vi "Segment File.vi"(8 "error in (no error)":errorcluster, 9 "current time in":timestamp, 10 "Current Bytes in":u64, 11 "Compiled.Settings":T1 {"Trigger Ref" format="%.0x"; "File Data"."Groups"."Channels"."Data Reference in" format="%.0x"}) -> (0 "error out":errorcluster, 1 "current time out":timestamp, 2 "Current Bytes out":u64, 3 "Boolean":bool)   [LabVIEW 2023, in "Embedded TDMS Logger Engine.lvlib"]
uses:
  Embedded TDMS Logger Engine.lvlib
  Shared/Compiled.Settings.ctl
  Shared/FileData.ctl
  Shared/GroupData.ctl
  Shared/Meta Data Item.ctl
  Shared/ChannelData.ctl
  <vilib>/NI VeriStand/Custom Device API/Data Reference.ctl
  Shared/SegmentOptions.ctl
  Shared/Embedded TDMS Logger Shared.lvlib
  <vilib>/NI VeriStand/Custom Device API/Custom Device API.lvlib
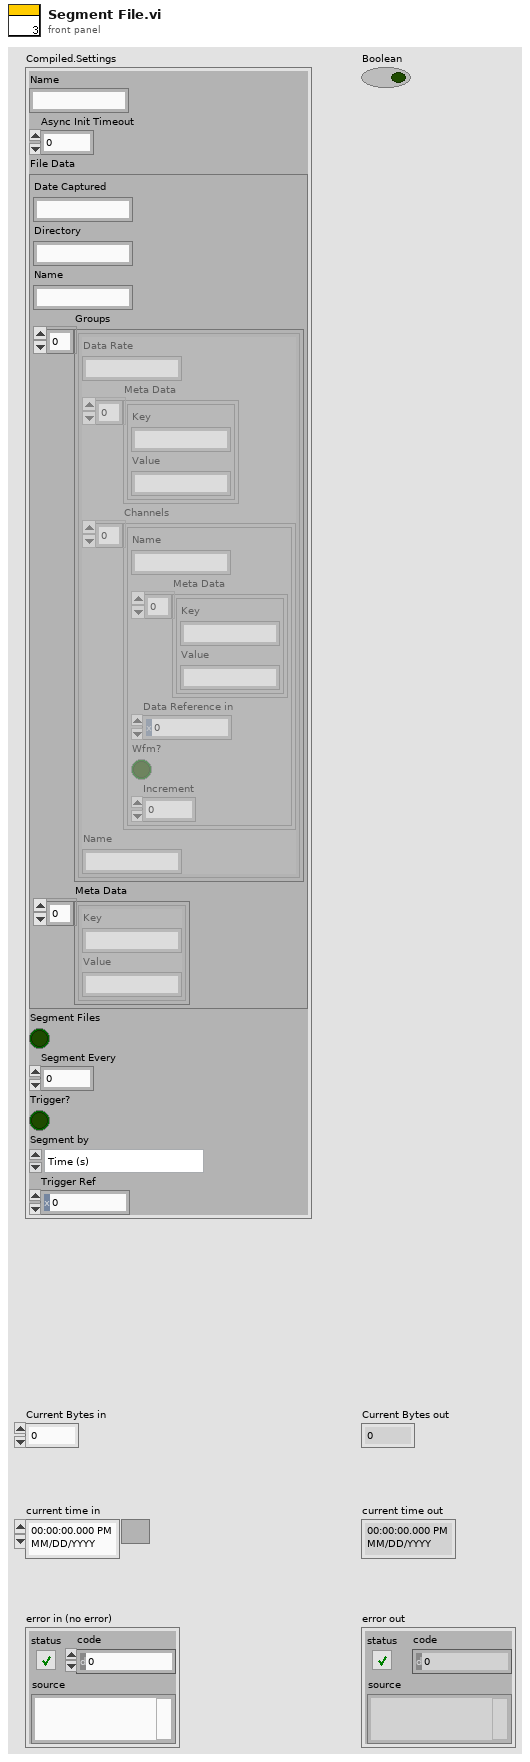
[diagram p1: front panel]
types:
  T1 = typedef "Embedded TDMS Logger Shared.lvlib/Compiled.Settings.ctl" = cluster{"Name":string, "Async Init Timeout":u16, "File Data":T2, "Segment Files":bool, "Segment Every":dbl, "Trigger?":bool, "Segment by":T7, "Trigger Ref":T6}
  T2 = typedef "Embedded TDMS Logger Shared.lvlib/FileData.ctl" = cluster{"Date Captured":string, "Directory":string, "Name":string, "Groups":T3[], "Meta Data":T4[]}
  T3 = typedef "Embedded TDMS Logger Shared.lvlib/GroupData.ctl" = cluster{"Data Rate":string, "Meta Data":T4[], "Channels":T5[], "Name":string}
  T4 = typedef "Embedded TDMS Logger Shared.lvlib/Meta Data Item.ctl" = cluster{"Key":string, "Value":string}
  T5 = typedef "Embedded TDMS Logger Shared.lvlib/ChannelData.ctl" = cluster{"Name":string, "Meta Data":T4[], "Data Reference":T6, "Wfm?":bool, "Increment":dbl}
  T6 = typedef "Custom Device API.lvlib/Data Reference.ctl" = i32
  T7 = typedef "SegmentOptions.ctl" = enum16{"Time (s)", "Size (MB)"}
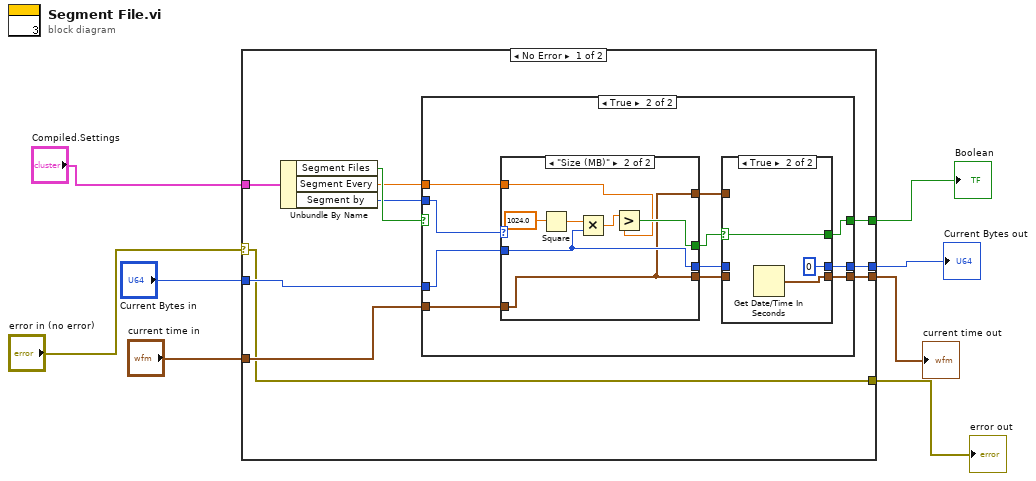
[diagram p0: block diagram]
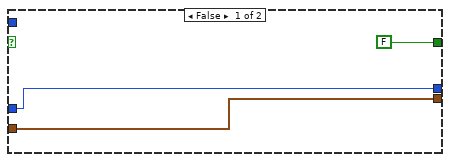
[diagram p2: hidden frame]
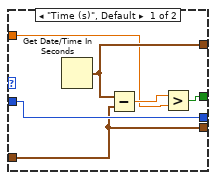
[diagram p4: hidden frame]
diagram:
  n1 = case shown="No Error" "error in (no error)" {
    selector: "error in (no error)" -> [w9 w52]
    tunnel: "Compiled.Settings" -> [w18 _]
    tunnel: [w16 _] -> w2
    tunnel: "Current Bytes in" -> [w15 w54]
    tunnel: "current time in" -> [w14 w53]
    tunnel: [w11 w54] -> w5
    tunnel: [w10 w53] -> w6
    tunnel: [w9 w52] -> w7
    frame No Error {
      n2 = Unbundle By Name(w18) -> ("Segment Files"=w17:bool, "Segment Every"=w12:dbl, "Segment by"=w13:T7)
      n3 = case shown="True" w17 {
        tunnel: [FALSE w27] -> w16
        tunnel: w15 -> [w20 w30]
        tunnel: w14 -> [w19 w29]
        tunnel: w13 -> [_ w32]
        tunnel: w12 -> [_ w31]
        tunnel: [w20 w26] -> w11
        tunnel: [w19 w24] -> w10
        frame False {
        }
        frame True {
          n4 = case shown="\"Size (MB)\"" w32 {
            tunnel: w31 -> [w39 w45]
            tunnel: w30 -> [w43 w48]
            tunnel: [w44 w49] -> w28
            tunnel: w29 -> [w42 w47]
            tunnel: [w43 w48] -> w25
            tunnel: [w42 w47] -> w23
            tunnel: [w41 w47] -> w22
            frame "Time (s)", Default {
              n5 = Get Date/Time In Seconds() -> (seconds since 1Jan1904=w41:timestamp)
              n6 = Subtract(x=w41, y=w42) -> (x-y=w40:dbl)
              n7 = Greater?(x=w40, y=w39) -> (0:w44:bool)
            }
            frame "Size (MB)" {
              n8 = Square(x=1024.0) -> (x^2=w50:dbl)
              n9 = Multiply(x=w50, y=w48) -> (x*y=w46:dbl)
              n10 = Greater?(x=w46, y=w45) -> (0:w49:bool)
            }
          }
          n11 = case shown="True" w28 {
            selector: w28 -> [w35 w38]
            tunnel: [w35 w38] -> w27
            tunnel: [w34 u64 0 ("Current Bytes")] -> w26
            tunnel: w25 -> [w34 _]
            tunnel: [w33 w36] -> w24
            tunnel: w23 -> [w33 _]
            tunnel: w22 -> [_ _]
            frame False {
            }
            frame True {
              n12 = Get Date/Time In Seconds() -> (seconds since 1Jan1904=w36:timestamp)
            }
          }
        }
      }
    }
    frame Error {
    }
  }
  "error out" <- w7
  "current time out" <- w6
  "Current Bytes out" <- w5
  "Boolean" <- w2
